vi "CLOSE.vi"(8 "error in (no error)":errorcluster, 11 "Database Ref In":T1) -> (0 "error out":errorcluster)   [LabVIEW 2018, in "MySQLTools.lvlib"]
uses:
  MySQLTools.lvlib
  <vilib>/addons/database/Connection.llb/Conn ObjectReference.ctl
  <vilib>/addons/database/NI_Database_API.lvlib
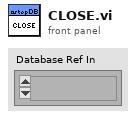
[diagram p1: front panel]
types:
  T1 = typedef "NI_Database_API.lvlib/Conn ObjectReference.ctl" = refnum<k1>
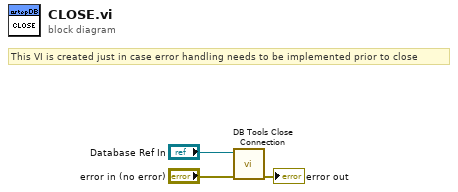
[diagram p0: block diagram]
diagram:
  # "This VI is created just in case error handling needs to be implemented prior to close"
  n1 = call <vilib>:"DB Tools Close Connection.vi"("error in (no error)"="error in (no error)", "connection reference"="Database Ref In") -> ("error out"=→"error out":errorcluster)  [unwired: 5 in]
